vi "KioskDemoRight.vi"() -> ()   [LabVIEW 2023]
doc: "DESCRIPTION\nGeneral Application \n\nVERSION\nD1:00\nFirst Release To customer\nDD/MM/YYYY\n\nTemplate D2:01\nMade lighter and simpler\n14-04-2020"
uses:
  SubVIs/Controls/SetupModeState.ctl
  <vilib>/event_ctls.llb/eventsource.ctl
  SubVIs/Controls/DisplayQCommand.ctl
  SubVIs/Controls/QueueCommand.ctl
  SubVIs/Controls/DisplayMessage.ctl
  SubVIs/utilities/Error/ErrorCommand.ctl
  SubVIs/Controls/Transition.ctl
  <vilib>/Utility/miscctls.llb/LVBoundsTypeDef.ctl
  SubVIs/Buttons/ButtonCommands.ctl
  SubVIs/Buttons/MenuType.ctl
  <vilib>/Utility/miscctls.llb/LVPositionTypeDef.ctl
  SubVIs/Controls/Tab.ctl
  SubVIs/Controls/StateMessage.ctl
  SubVIs/Error/ErrorMessage.ctl
  SubVIs/utilities/Config/System Config Data Manager Parameter.ctl
  SubVIs/utilities/Config/ConfigCommand.ctl
panel:
  out "Selector ref out":refnum<vi>
  in  "Tab Control 2":enum32{"Page 3"}(tab)
  out "BGND ref out":refnum<vi>
  in  "exit":bool
  out "Application Directory":path
  in  "ButtonsMenu":enum32{"Page 1"}(tab)
  out "SubmenuVisible":bool
  out "State":T1=enum."Initialising"
  out "UI Output":string
  out "Menu Output":string
  in  "Stop":bool
  in  "Source":T2 items=["LabVIEW UI"=0, "ActiveX"=1, "User Event"=25]
  in  "Start":bool
  out "ErrorHandlingLoop":i32
  out "StateMachineLoop":i32
  out "UILoop":i32
  out "EventLoop":i32
  in  "Main Screen Tabs":enum32{"Main Screen"}(tab)
  out "Tab Control":T3(tab)
  in  "Error Loop":enum16{"Event Loop", "UI Q Loop", "State Loop"}(ring)
  in  "Generate Error":bool
  out "EngMode?":bool
  in  "Enter Password":string
  out "ConfigdB path":path
  in  "Home Button":bool
  in  "ErrorLog":bool
  in  "Clear Alarm":bool
  in  "ErrorLog":i32(listbox)
  out "Error":string
  out "ErrorIndicator":bool
  in  "ViewError":bool
  out "Version":string
  out "Time":string
  out "Status":string
  # "GenAppMain"
  # "Move to right and change sub menu"
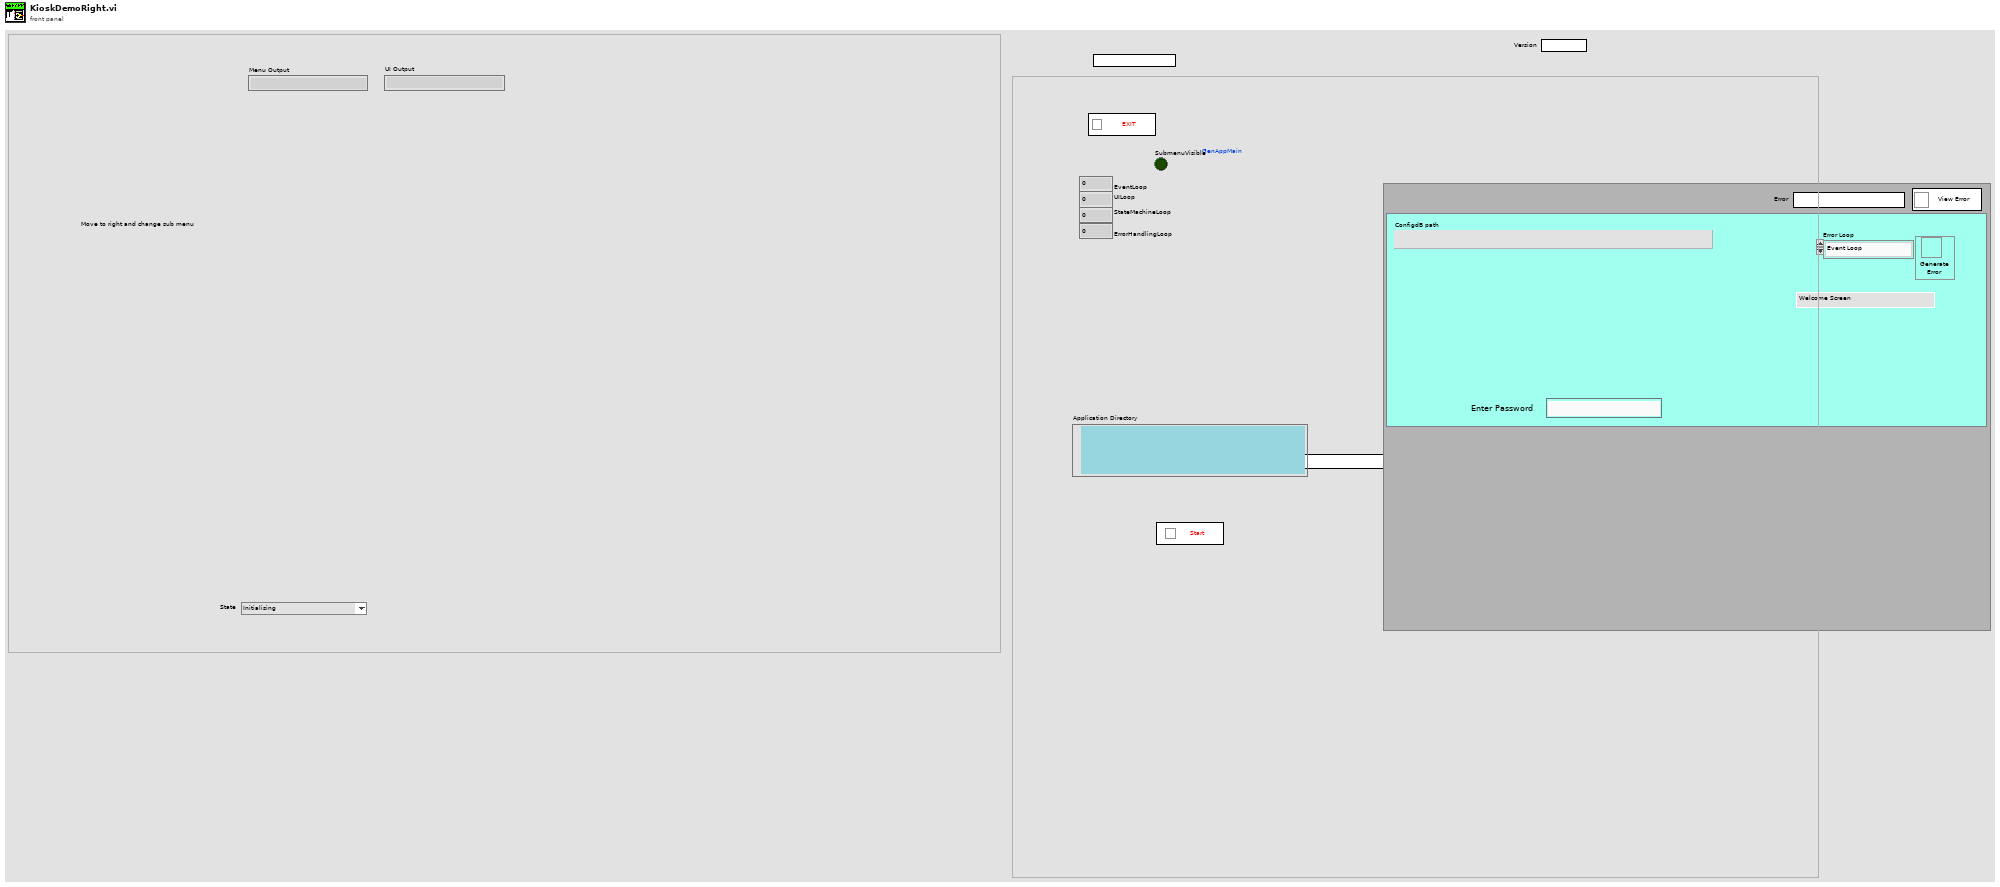
[diagram p1: front panel]
types:
  T1 = typedef "SetupModeState.ctl" = enum16{"No State - Error", "Initialising", "Idling", "Running", "Sorting Menu", "Resetting Menu", "Sorting Submenu", "Loading UI", "Erroring", "Exiting"}
  T2 = typedef "eventsource.ctl" = u32
  T3 = enum32{"Welcome Screen", "Eng Set Up", "Oppo Run Screen", "Eng Run Screen", "Test Report Screen", "Error"}
  T4 = typedef "DisplayQCommand.ctl" = enum16{"No Command - Error", "Initialise", "Get Q Reference", "Add Item to Bottom", "Add Item to Top", "Flush Q", "Dequeue", "Peek Next Element", "Close"}
  T5 = typedef "QueueCommand.ctl" = enum16{"No Command - Error", "Initialise", "Add to Bottom", "Add To Top", "Get Ref", "Close"}
  T6 = typedef "LVBoundsTypeDef.ctl" = cluster{"Width":u32, "Height":u32}
  T7 = typedef "ErrorCommand.ctl" = enum16{"No Command - Error", "Set to Dev Mode", "Set To Released Mode", "Set Error", "Log Error", "Throw Error", "Log & Throw Error", "Set Error Timed"}
  T8 = enum32{"invalid app kind", "Development System", "Run Time System", "Student Edition", "Embedded LabVIEW", "Evaluation", "Custom"}
  T9 = typedef "LVPositionTypeDef.ctl" = cluster{"Left":i32, "Top":i32}
  T10 = typedef "StateMessage.ctl" = cluster{"Transition":T11, "variant":variant}
  T11 = typedef "Transition.ctl" = enum16{"No Transition - Error", "Initialise", "Login", "Authenticate", "Log on Fail", "Login Success", "Logout", "Generate Error", "Start", "Stop", "Menu Button Pressed", "UI Button Pressed", "Exit"}
  T12 = typedef "DisplayMessage.ctl" = enum16{"No Message - Ignore", "Display Message", "Set Tab", "Set Status", "Add Error Message", "Clear Error History", "Generate Error", "Set Idling Display", "Set Running Display", "Set Subpanel Output", "Stop"}
  T13 = typedef "ErrorMessage.ctl" = enum16{"No Message - Ignore", "Display Message", "Stop"}
  T14 = typedef "ConfigCommand.ctl" = enum16{"No Command - Error", "Initialise Config SQLite", "Save Config", "Get Key", "Set Key", "Update Key", "Get Latest Config Data", "Get Config Data for Version", "Get Default Config Data"}
  T15 = typedef "System Config Data Manager Parameter.ctl" = enum16{"Eng Password", "DSN Connection", "User Password", "RunStatus", "InitialDataPath", "helpFilePath", "ErrorFilepath", "DatalogPath", "Hello"}
  T16 = typedef "Tab.ctl" = enum32{"Welcome Screen", "Eng Set Up", "Oppo Run Screen", "Eng Run Screen", "Test Report Screen", "Error"}
  T17 = typedef "lveventtype.ctl" = enum32{"Null", "Timeout", "Annotation Menu Selection", "Annotation Menu Selection?", "App Instance Close", "App Instance Close?", "Autoscale Range Change", "Bookmark Info Change", "Cell Edit", "Cell Edit?", "Cursor Grab", "Cursor Grab?", "Cursor Menu Selection", "Cursor Menu Selection?", "Cursor Move", "Cursor Release", "Data Change", "Direction Change", "Display State Change", "Drag Ended", "Drag Enter", "Drag Leave", "Drag Over", "Drag Source Update", "Drag Starting", "Drag Starting?", "Drop", "Exec State Change", "Key Down", "Key Down?", "Key Repeat", "Key Repeat?", "Key Up", "Listbox Double Click", "Menu Activation?", "Menu Selection (App)", "Menu Selection? (App)", "Menu Selection (User)", "Mouse Down", "Mouse Down?", "Mouse Enter", "Mouse Leave", "Mouse Move", "Mouse Up", "Mouse Wheel", "NI Security User Change (App)", "Pane Size", "Panel Close", "Panel Close?", "Panel Resize", "Plot Attribute Change", "Scale Range Change", "Shortcut Menu Activation?", "Shortcut Menu Selection (App)", "Shortcut Menu Selection? (App)", "Shortcut Menu Selection (User)", "Tree Double Click", "Tree Drag", "Tree Drag?", "Tree Drop", "Tree Drop?", "Tree Item Close", "Tree Item Close?", "Tree Item Open", "Tree Item Open?", "User Event", "Value Change"}
  T18 = typedef "MenuType.ctl" = enum16{"Main", "Simulation", "ME", "SF", "User Utilities", "Dev Tools"}
  T19 = typedef "ButtonCommands.ctl" = enum16{"No Command - Error", "Load Buttons", "Remove Buttons", "Get User Event"}
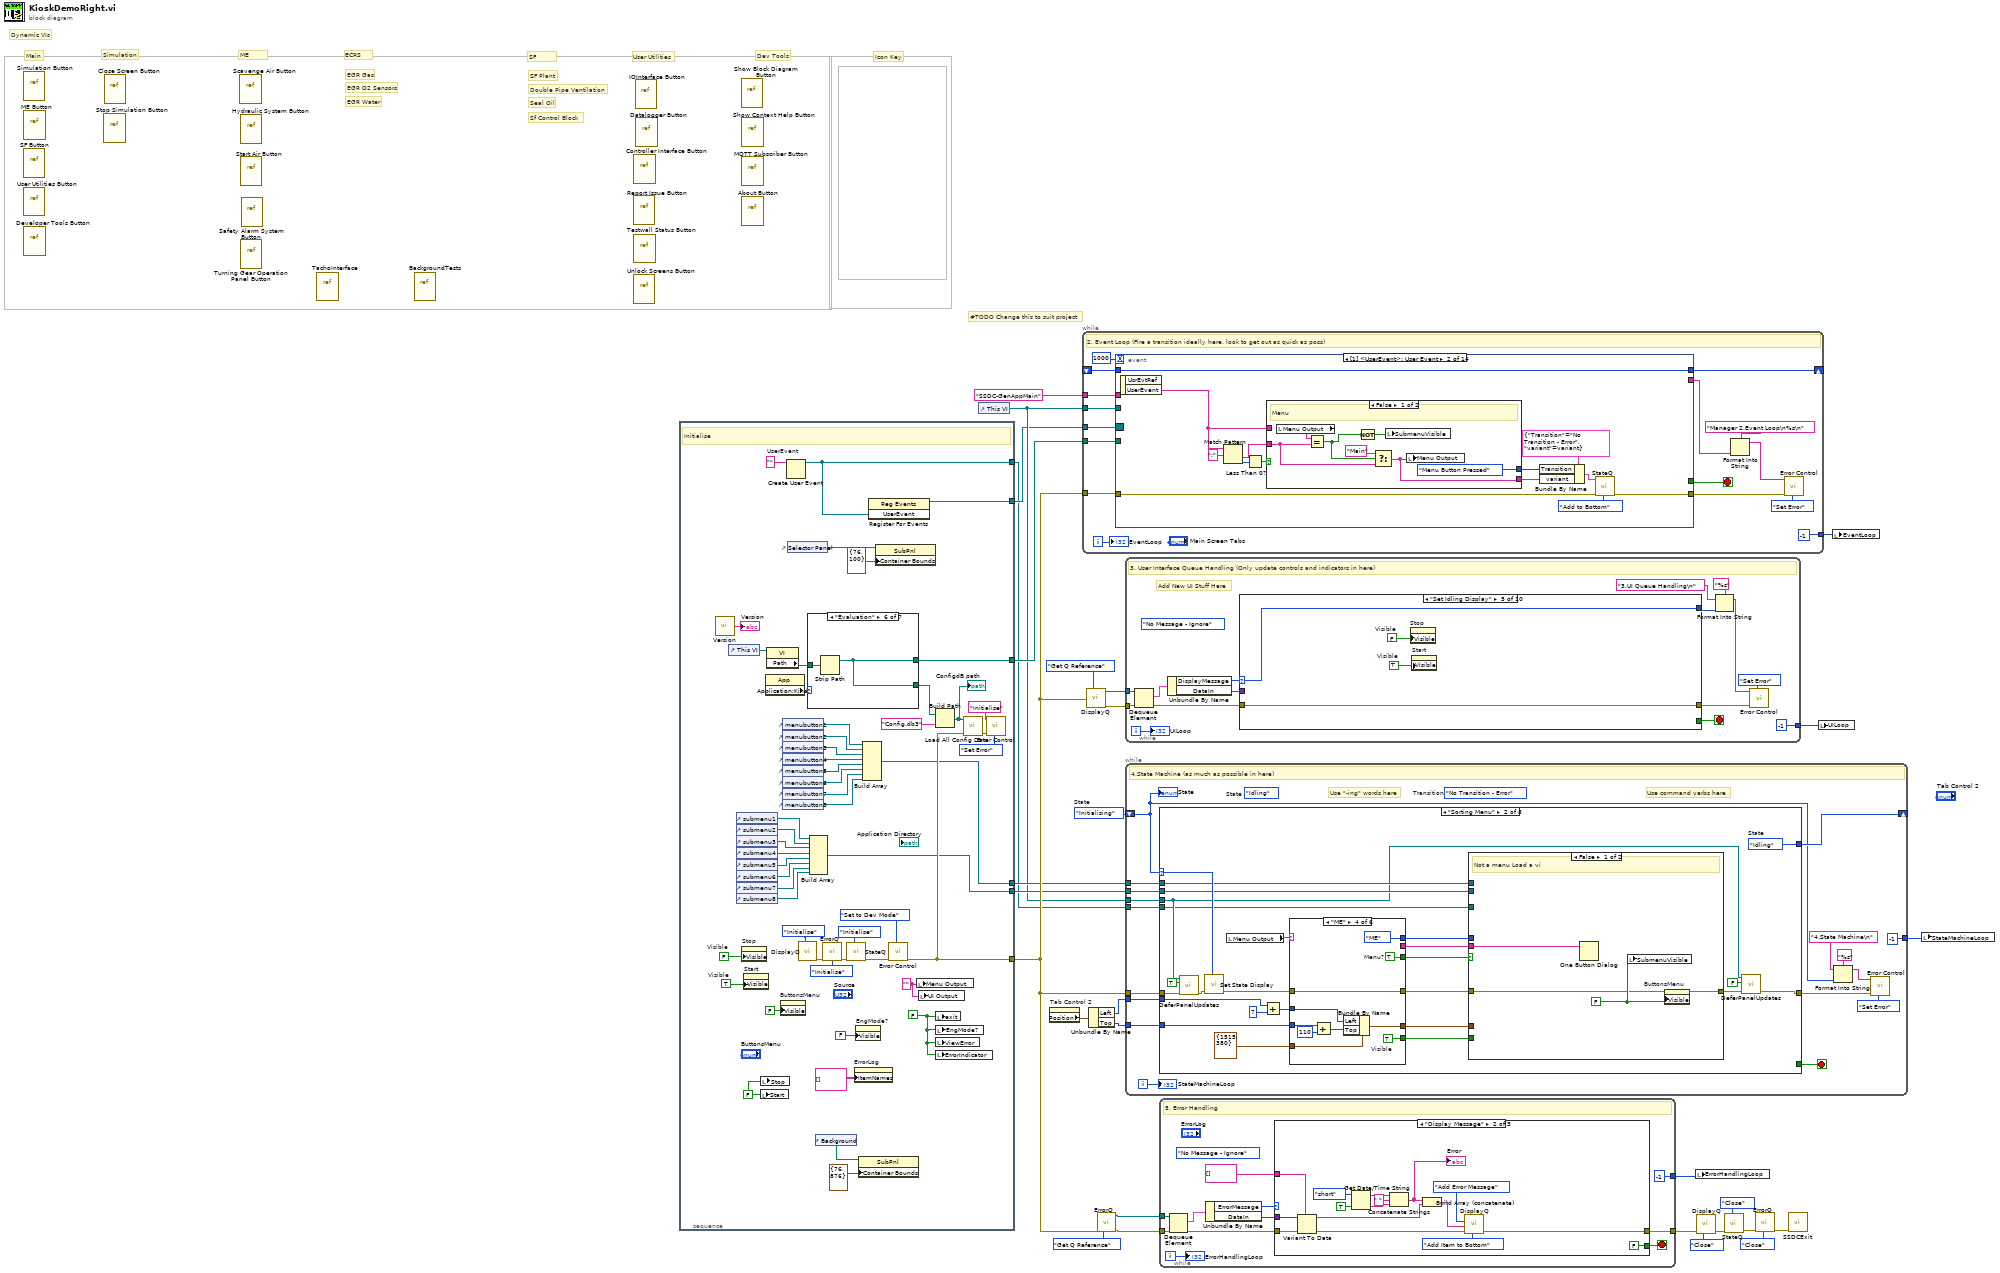
[diagram p0: block diagram]
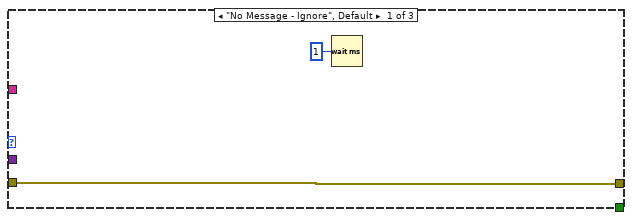
[diagram p2: hidden frame]
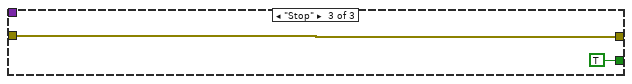
[diagram p3: hidden frame]
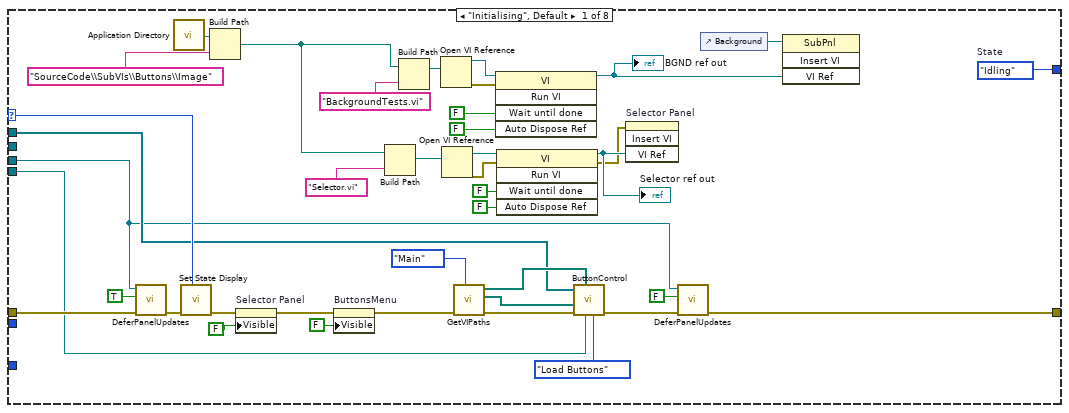
[diagram p4: hidden frame]
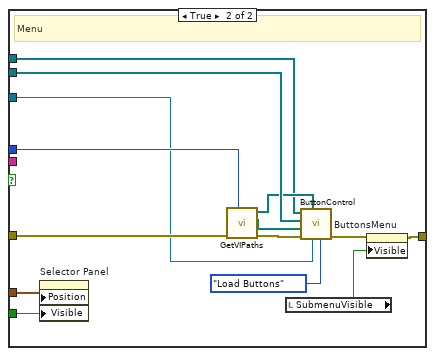
[diagram p5: hidden frame]
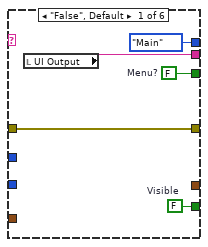
[diagram p6: hidden frame]
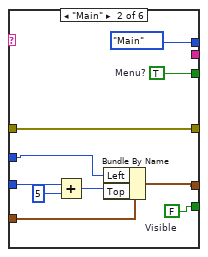
[diagram p7: hidden frame]
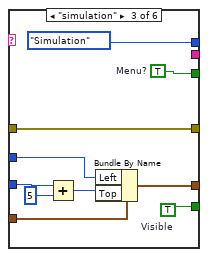
[diagram p8: hidden frame]
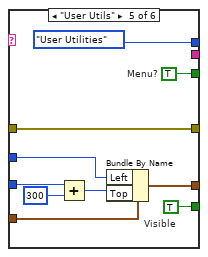
[diagram p9: hidden frame]
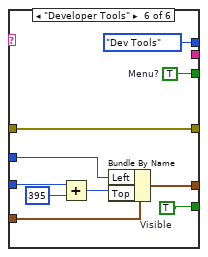
[diagram p10: hidden frame]
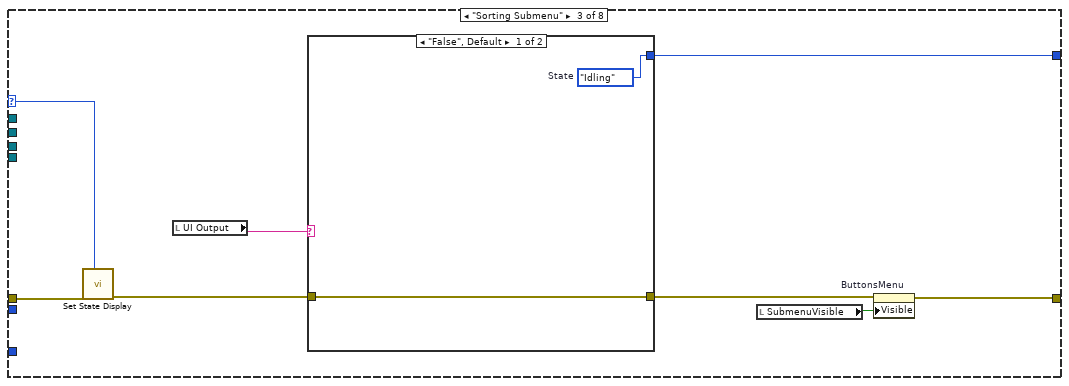
[diagram p11: hidden frame]
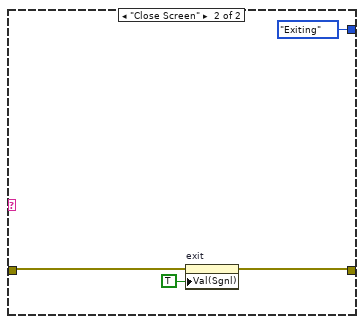
[diagram p12: hidden frame]
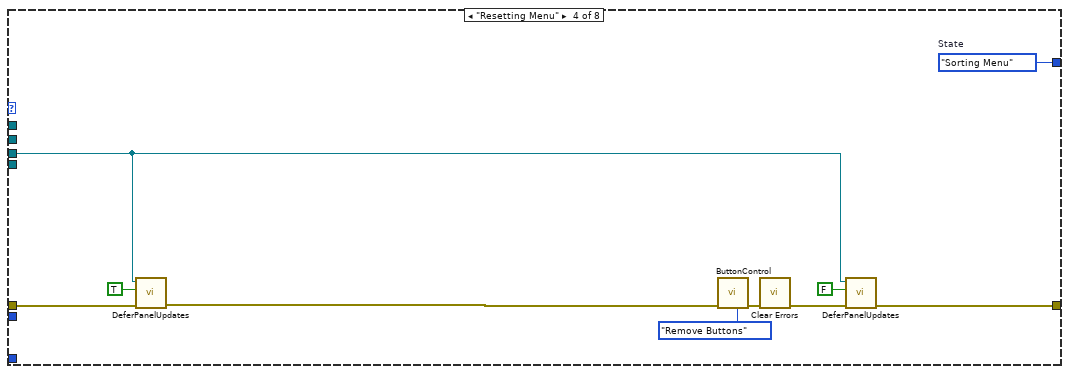
[diagram p13: hidden frame]
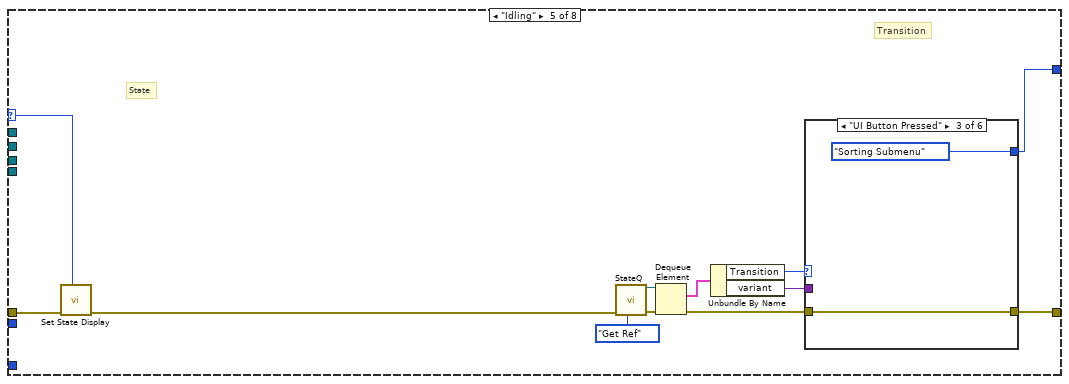
[diagram p14: hidden frame]
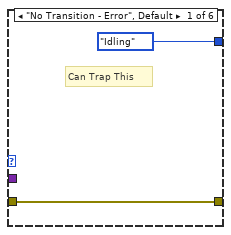
[diagram p15: hidden frame]
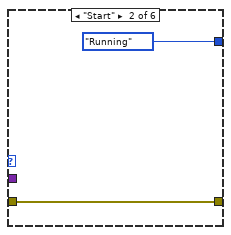
[diagram p16: hidden frame]
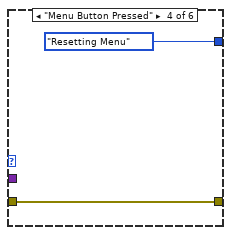
[diagram p17: hidden frame]
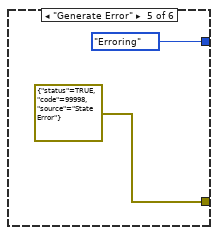
[diagram p18: hidden frame]
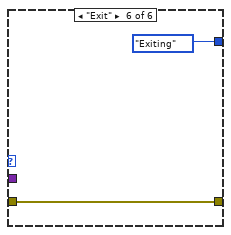
[diagram p19: hidden frame]
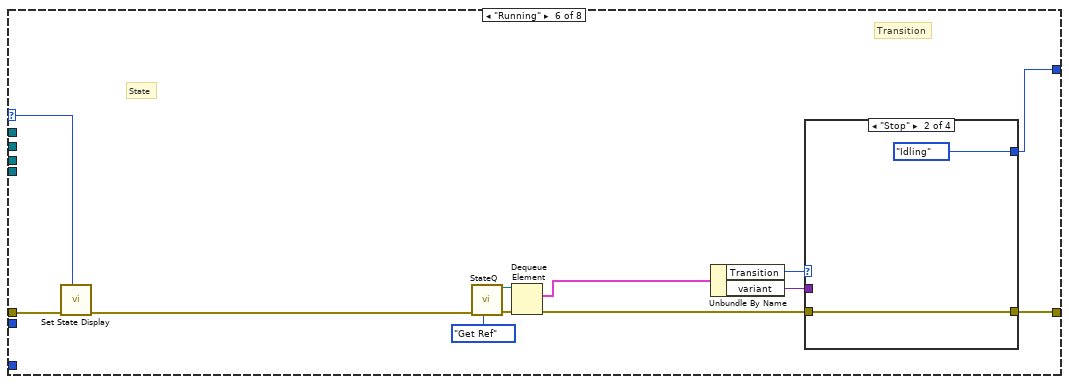
[diagram p20: hidden frame]
diagram:
  w29 = SetupModeState."Initialising"  # State
  # "Sf Control Block"
  # "Seal Oil"
  # "Double Pipe Ventilation"
  # "SF Plant"
  # "SF"
  # "EGR Water"
  # "EGR O2 Sensors"
  # "EGR Gas"
  # "ECRS"
  # "Dev Tools"
  # "User Utilities"
  # "Main"
  # "Simulation"
  # "ME"
  # "Dynamic VIs"
  # "#TODO Change this to suit project"
  # "Icon Key"
  n1 = vi-ref "Simulation Button.vi"() -> ()  [unwired: 1 out]
  n2 = vi-ref "SF Button.vi"() -> ()  [unwired: 1 out]
  n3 = vi-ref "User Utilities Button.vi"() -> ()  [unwired: 1 out]
  n4 = vi-ref "ME Button.vi"() -> ()  [unwired: 1 out]
  n5 = vi-ref "Developer Tools Button.vi"() -> ()  [unwired: 1 out]
  n6 = vi-ref "Stop Simulation Button.vi"() -> ()  [unwired: 1 out]
  n7 = vi-ref "Close Screen Button.vi"() -> ()  [unwired: 1 out]
  n8 = vi-ref "Scavenge Air Button.vi"() -> ()  [unwired: 1 out]
  n9 = vi-ref "Hydraulic System Button.vi"() -> ()  [unwired: 1 out]
  n10 = vi-ref "Start Air Button.vi"() -> ()  [unwired: 1 out]
  n11 = vi-ref "Turning Gear Operation Panel Button.vi"() -> ()  [unwired: 1 out]
  n12 = vi-ref "Safety Alarm System Button.vi"() -> ()  [unwired: 1 out]
  n13 = vi-ref "TachoInterface.vi"() -> ()  [unwired: 1 out]
  n14 = vi-ref "BackgroundTests.vi"() -> ()  [unwired: 1 out]
  n15 = vi-ref "Report Issue Button.vi"() -> ()  [unwired: 1 out]
  n16 = vi-ref "Unlock Screens Button.vi"() -> ()  [unwired: 1 out]
  n17 = vi-ref "Controller Interface Button.vi"() -> ()  [unwired: 1 out]
  n18 = vi-ref "Testwall Status Button.vi"() -> ()  [unwired: 1 out]
  n19 = vi-ref "IOInterface Button.vi"() -> ()  [unwired: 1 out]
  n20 = vi-ref "Datalogger Button.vi"() -> ()  [unwired: 1 out]
  n21 = stacked-sequence "1. Initialisation" {
    tunnel: [w60] -> w16
    tunnel: [w65] -> w24
    tunnel: [w49] -> w8
    tunnel: [w41] -> w7
    tunnel: [w35] -> w1
    tunnel: [w34] -> w5
    frame #0 {
      w36 = ""  # UserEvent
      w39 = "" ("Menu Output")
      w58 = FALSE  # Visible
      w57 = TRUE  # Visible
      w63 = FALSE ("Stopped")
      w59 = FALSE ("Start")
      # "Initialise"
      n22 = call "Version.vi"() -> ("Version"=→"Version":string)  [unwired: 5 in]
      n23 = control-ref of="This VI"() -> (w76:refnum<vi>)
      n24 = control-ref of="submenu1"() -> (w48:refnum<vi>)
      n25 = control-ref of="submenu2"() -> (w47:refnum<vi>)
      n26 = control-ref of="submenu3"() -> (w46:refnum<vi>)
      n27 = control-ref of="submenu4"() -> (w45:refnum<vi>)
      n28 = control-ref of="submenu5"() -> (w44:refnum<vi>)
      n29 = control-ref of="submenu6"() -> (w43:refnum<vi>)
      n30 = control-ref of="submenu7"() -> (w42:refnum<vi>)
      n31 = control-ref of="submenu8"() -> (w38:refnum<vi>)
      n32 = property on="Stop" class="Bool (strict)"("Visible"=w58) -> ()  [unwired: 2 in, 2 out]
      n33 = property on="Start" class="Bool (strict)"("Visible"=w57) -> ()  [unwired: 2 in, 2 out]
      n34 = local write "Start"(w59) -> ()
      n35 = local write "Stop"(w59) -> ()
      n36 = property class="App"() -> ("Application:Kind"=w75:T8)  [unwired: 2 in, 2 out]
      n37 = property class="VI"(reference=w76) -> ("Path"=w77:path)  [unwired: 1 in, 2 out]
      n38 = property on="ButtonsMenu" class="TabCtl (strict)"("Visible"=FALSE) -> ()  [unwired: 2 in, 2 out]
      n39 = control-ref of="menubutton1"() -> (w51:refnum<vi>)
      n40 = control-ref of="menubutton2"() -> (w50:refnum<vi>)
      n41 = control-ref of="menubutton3"() -> (w56:refnum<vi>)
      n42 = control-ref of="menubutton4"() -> (w55:refnum<vi>)
      n43 = control-ref of="menubutton5"() -> (w54:refnum<vi>)
      n44 = control-ref of="menubutton6"() -> (w53:refnum<vi>)
      n45 = control-ref of="menubutton7"() -> (w52:refnum<vi>)
      n46 = control-ref of="menubutton8"() -> (w40:refnum<vi>)
      n47 = Create User Event(user event datatype=w36) -> (user event=w35:refnum<user-event>)  [unwired: 1 in, 1 out]
      n48 = control-ref of="Selector Panel"() -> (w31:refnum<vi>)
      n49 = call "DisplayQ.vi"("command"=DisplayQCommand."Initialise") -> ("error out"=w70:errorcluster)  [unwired: 4 in, 3 out]
      n50 = case shown="\"Evaluation\"" w75 {
        tunnel: w77 -> [w82 w84 w88 w91 w93 w95 w97]
        tunnel: [w82 w83 w87 w90 w92 w94 w96] -> w66
        tunnel: [w82 w83 w85 w90 w92 w94 w96] -> w65
        frame "invalid app kind", Default {
        }
        frame "Development System" {
          n51 = Strip Path(path=w84) -> (stripped path=w83:path)  [unwired: 1 out]
        }
        frame "Run Time System" {
          n52 = Strip Path(path=w88) -> (stripped path=w89:path)  [unwired: 1 out]
          n53 = Strip Path(path=w89) -> (stripped path=w85:path)  [unwired: 1 out]
          n54 = Build Path(base path=w85, name or relative path="data") -> (appended path=w87:path)
        }
        frame "Student Edition" {
          n55 = Strip Path(path=w91) -> (stripped path=w90:path)  [unwired: 1 out]
        }
        frame "Embedded LabVIEW" {
          n56 = Strip Path(path=w93) -> (stripped path=w92:path)  [unwired: 1 out]
        }
        frame "Evaluation" {
          n57 = Strip Path(path=w95) -> (stripped path=w94:path)  [unwired: 1 out]
        }
        frame "Custom" {
          n58 = Strip Path(path=w97) -> (stripped path=w96:path)  [unwired: 1 out]
        }
      }
      n59 = Build Array(w48, w47, w46, w45, w44, w43, w42, w38) -> (w41:refnum<vi>[])
      n60 = control-ref of="Background"() -> (w33:refnum<vi>)
      n61 = call "ErrorQ.vi"("command"=DisplayQCommand."Initialise", "error in (no error)"=w70) -> ("error out"=w71:errorcluster)  [unwired: 3 in, 3 out]
      n62 = call "StateQ.vi"("QueueCommand"=QueueCommand."Initialise", "error in (no error)"=w71) -> ("error out"=w61:errorcluster)  [unwired: 5 in, 1 out]
      n63 = property on="ErrorLog" class="MCListbox (strict)"("ItemNames"=string[][] [] ("Item Names")) -> ()  [unwired: 2 in, 2 out]
      n64 = property on="EngMode?" class="Bool (strict)"("Visible"=FALSE) -> ()  [unwired: 2 in, 2 out]
      n65 = property class="SubPnl"(reference=w33, "Container Bounds"=T6 {"Width"=76, "Height"=876}) -> ()  [unwired: 1 in, 2 out]
      n66 = Build Array(w51, w50, w56, w55, w54, w53, w52, w40) -> (w49:refnum<vi>[])
      n67 = register-events(w35) -> (reference out=w34:refnum<event-registration>)  [unwired: 2 in, 1 out]
      n68 = property class="SubPnl"(reference=w31, "Container Bounds"=T6 {"Width"=76, "Height"=100}) -> ()  [unwired: 1 in, 2 out]
      n69 = call "Error Control.vi"("Command"=ErrorCommand."Set to Dev Mode", "error in (no error)"=w61) -> ("error out"=w60:errorcluster)  [unwired: 6 in]
      n70 = local write "Menu Output"(w39) -> ()
      n71 = local write "UI Output"(w39) -> ()
      n72 = local write "exit"(w63) -> ()
      n73 = local write "ViewError"(w63) -> ()
      n74 = local write "ErrorIndicator"(w63) -> ()
      n75 = Build Path(base path=w66, name or relative path="Config.db3") -> (appended path=w78:path)
      "ConfigdB path" <- w78
      n76 = local write "EngMode?"(w63) -> ()
      n77 = call "Load All Config Data.vi"("error in (no error)"=w60, "path"=w78) -> ("error out"=w68:errorcluster)  [unwired: 5 in]
      n78 = call "Error Control.vi"("Command"=ErrorCommand."Set Error", "error in (no error)"=w68, "Source"="Initialise") -> ()  [unwired: 5 in, 1 out]
    }
  }
  n79 = vi-ref "Show Block Diagram Button.vi"() -> ()  [unwired: 1 out]
  n80 = vi-ref "Show Context Help Button.vi"() -> ()  [unwired: 1 out]
  n81 = vi-ref "MQTT Subscriber Button.vi"() -> ()  [unwired: 1 out]
  n82 = vi-ref "About Button.vi"() -> ()  [unwired: 1 out]
  n83 = control-ref of="This VI"() -> (w6:refnum<vi>)
  n84 = property on="Tab Control 2" class="TabCtl (strict)"() -> ("Position"=w4:T9)  [unwired: 2 in, 2 out]
  n85 = while "2. Event Loop" {
    tunnel: w16 -> [w110]
    shift-right: [w107] -> _
    shift-left: _ -> [w106]
    tunnel: w6 -> [w105]
    tunnel: [-1 ("ErrorHandlingLoop")] -> w25
    tunnel: w24 -> [w103]
    tunnel: "SSDC-GenAppMain" ("name or relative path") -> [w102]
    tunnel: w5 -> [w98]
    i -> [w113]
    stop <- w112 stop-if-true
    # "2. Event Loop (Fire a transition ideally here, look to get out as quick as poss)"
    n86 = event shown="[1] <UserEvent>: User Event" {
      selector: w98 -> [_ _ _ _ _ _ _ _ _ _ _ _ _ _]
      dyn-events: _ -> [_ _ _ _ _ _ _ _ _ _ _ _ _ _]
      timeout: 1000 -> [_ _ _ _ _ _ _ _ _ _ _ _ _ _]
      tunnel: [_ _ FALSE ("STOP?") _ TRUE ("STOP?") _ _ _ w219 _ _ _ _ _] -> w112
      tunnel: w110 -> [_ w122 w145 _ _ w177 w192 _ w216 w236 w254 w267 w290 _]
      tunnel: [_ w121 w145 _ _ w176 w191 _ w215 w235 w253 w266 w289 _] -> w108
      tunnel: ["Timeout" _ "Panel Close?" ("Event") w149 w156 w173 w187 w201 w210 w228 w247 w260 w283 w302] -> w99
      tunnel: [w116 w133 w144 w154 w159 w180 w194 w204 w218 w231 w252 w263 w291 w306] -> w107
      tunnel: w106 -> [w116 w133 w144 w154 w159 w180 w194 w204 w218 _ w252 w263 w291 w306]
      tunnel: w105 -> [_ _ _ _ _ _ _ _ w217 _ _ _ _ w305]
      tunnel: w103 -> [_ _ _ _ _ _ _ _ w214 _ _ _ _ _]
      tunnel: w102 -> [_ _ _ _ _ _ _ _ _ _ _ _ _ _]
      event Timeout {
        n87 = event-data() -> ()  [unwired: 1 in, 1 out]
        n88 = Get Date/Time String(want seconds? (F)=TRUE) -> (date string=w119:string, time string=w118:string)  [unwired: 2 in]
        n89 = Concatenate Strings(w119, " " ("string"), w118) -> (→"Time":string)
      }
      event User Event {
        n90 = event-data() -> ("UserEvent"=w123:string)  [unwired: 1 in, 1 out]
        n91 = Match Pattern(string=w123, regular expression=":") -> (after substring=w132:string, offset past match=w128:i32)  [unwired: 1 in, 2 out]
        n92 = Less Than 0?(x=w128) -> (x < 0?=w129:bool)
        n93 = case shown="False" w129 {
          tunnel: w132 -> [w137 _]
          tunnel: [Transition."Menu Button Pressed" ("Transition") Transition."UI Button Pressed" ("Transition")] -> w130
          tunnel: [w134 w141] -> w131
          tunnel: w123 -> [_ w141]
          frame False {
            # "Menu"
            n94 = local read "Menu Output"() -> (w139:string)
            n95 = Equal?(x=w139, y=w137) -> (x = y?=w136:bool)
            n96 = Not(x=w136) -> (.not. x?=w135:bool)
            n97 = Select(t="Main", s=w136, f=w137) -> (s? t:f=w134:string)
            n98 = local write "SubmenuVisible"(w135) -> ()
            n99 = local write "Menu Output"(w134) -> ()
          }
          frame True {
            # "UI"
            n100 = local write "UI Output"(w141) -> ()
          }
        }
        n101 = Bundle By Name(cluster=T10 {"Transition"=enum."No Transition - Error", "variant"=variant} ("output cluster"), "Transition"=w130, "variant"=w131) -> (w127:T10)
        n102 = call "StateQ.vi"("QueueCommand"=QueueCommand."Add to Bottom", "error in (no error)"=w122, "output cluster"=w127) -> ("error out"=w121:errorcluster)  [unwired: 4 in, 1 out]
      }
      event Panel Close? {
        n103 = event-data() -> ()  [unwired: 1 in, 1 out]
        n104 = property on="exit" class="Bool (strict)"("Val(Sgnl)"=TRUE ("Value (Signaling)")) -> ()  [unwired: 2 in, 2 out]
        n105 = event-data("Discard?"=TRUE) -> ()  [unwired: 1 in, 1 out]
      }
      event "ErrorLog": Value Change {
        n106 = event-data() -> ("CtlRef"=w151:refnum<vi>, "Type"=w150:T17)  [unwired: 1 in]
        n107 = call "CreateEventString.vi"("Type in"=w150, "Ctl Refnum"=w151) -> ("Event"=w149:string)  [unwired: 9 in]
        n108 = case shown="True" "ErrorLog" {
          tunnel: [_ FALSE] -> w152
          frame False {
          }
          frame True {
            n109 = call "ErrorLogDialog.vi"() -> ()  [unwired: 11 in, 1 out]
          }
        }
        n110 = local write "ErrorLog"(w152) -> ()
      }
      event "exit": Value Change {
        n111 = event-data() -> ("CtlRef"=w158:refnum<vi>, "Type"=w157:T17)  [unwired: 1 in]
        n112 = local write "Start"(FALSE ("Start")) -> ()
        n113 = call "CreateEventString.vi"("Type in"=w157, "Ctl Refnum"=w158) -> ("Event"=w156:string)  [unwired: 9 in]
        n114 = stacked-sequence {
          tunnel: [_ FALSE] -> w160
          frame #0 {
            n115 = call "StateQ.vi"("QueueCommand"=QueueCommand."Add To Top", "output cluster"=T10 {"Transition"=enum."Exit", "variant"=variant}) -> ("error out"=w167:errorcluster)  [unwired: 5 in, 1 out]
            n116 = call "ErrorQ.vi"("command"=DisplayQCommand."Add Item to Top", "error in (no error)"=w167, "ErrorMessage"=ErrorMessage."Stop") -> ("error out"=w164:errorcluster)  [unwired: 2 in, 3 out]
            n117 = call "DisplayQ.vi"("command"=DisplayQCommand."Add Item to Top", "error in (no error)"=w164, "DisplayMessage"=DisplayMessage."Stop") -> ()  [unwired: 2 in, 4 out]
          }
          frame #1 {
            n118 = Wait (ms)(milliseconds to wait=u32 500) -> ()  [unwired: 1 out]
          }
        }
        n119 = local write "exit"(w160) -> ()
      }
      event "Start": Value Change {
        n120 = event-data() -> ("CtlRef"=w175:refnum<vi>, "Type"=w174:T17)  [unwired: 1 in]
        n121 = call "CreateEventString.vi"("Type in"=w174, "Ctl Refnum"=w175) -> ("Event"=w173:string)  [unwired: 9 in]
        n122 = case shown="True" "Start" {
          tunnel: [_ FALSE ("Start")] -> w178
          tunnel: w177 -> [w181 w183]
          tunnel: [w181 w182] -> w176
          frame False {
          }
          frame True {
            n123 = call "StateQ.vi"("QueueCommand"=QueueCommand."Add To Top", "error in (no error)"=w183, "output cluster"=T10 {"Transition"=enum."Start", "variant"=variant}) -> ("error out"=w182:errorcluster)  [unwired: 4 in, 1 out]
          }
        }
        n124 = local write "Start"(w178) -> ()
      }
      event "Stop": Value Change {
        n125 = event-data() -> ("CtlRef"=w189:refnum<vi>, "Type"=w188:T17)  [unwired: 1 in]
        n126 = call "CreateEventString.vi"("Type in"=w188, "Ctl Refnum"=w189) -> ("Event"=w187:string)  [unwired: 9 in]
        n127 = case shown="True" "Stop" {
          tunnel: [_ FALSE ("Start")] -> w193
          tunnel: w192 -> [w195 w197]
          tunnel: [w195 w196] -> w191
          frame False {
          }
          frame True {
            n128 = call "StateQ.vi"("QueueCommand"=QueueCommand."Add To Top", "error in (no error)"=w197, "output cluster"=T10 {"Transition"=enum."Stop", "variant"=variant}) -> ("error out"=w196:errorcluster)  [unwired: 4 in, 1 out]
          }
        }
        n129 = local write "Stop"(w193) -> ()
      }
      event "Enter Password": Value Change {
        n130 = event-data() -> ("CtlRef"=w203:refnum<vi>, "Type"=w202:T17)  [unwired: 1 in]
        n131 = call "CreateEventString.vi"("Type in"=w202, "Ctl Refnum"=w203) -> ("Event"=w201:string)  [unwired: 9 in]
        n132 = call "SQLiteConfig.vi"("ConfigCommand"=ConfigCommand."Get Key", "Parameter"=System_Config_Data_Manager_Parameter."Eng Password") -> ("KeyData"=w205:string)  [unwired: 3 in, 3 out]
        n133 = Equal?(x=w205, y="Enter Password") -> (x = y?=w209:bool)
        "EngMode?" <- w209
        n134 = property on="EngMode?" class="Bool (strict)"("Visible"=w209) -> ()  [unwired: 2 in, 2 out]
      }
      event Menu Selection (User) {
        n135 = event-data() -> ("Type"=w212:T17, "ItemTag"=w211:string)  [unwired: 1 in]
        n136 = Format Into String(format string="\"Menu\":%s:%s", w212, w211) -> (resulting string=w210:string)  [unwired: 2 in, 1 out]
        n137 = case shown="\"About\"" w211 {
          tunnel: [_ FALSE _ _] -> w219
          tunnel: w217 -> [_ _ _ w227]
          tunnel: w216 -> [w220 w221 w224 w225]
          tunnel: [w220 w221 w224 w225] -> w215
          tunnel: w214 -> [_ _ _ _]
          frame "False", Default {
          }
          frame "Exit" {
            n138 = property on="exit" class="Bool (strict)"("Val(Sgnl)"=TRUE ("Value (Signaling)")) -> ()  [unwired: 2 in, 2 out]
          }
          frame "Configuration" {
            n139 = call "ConfigSQLiteSettingDialog.vi"() -> ()  [unwired: 1 in]
          }
          frame "About" {
            n140 = property class="VI"(reference=w227) -> ("Description"=w226:string)  [unwired: 1 in, 2 out]
            n141 = call "AboutScreen.vi"("Version Info. In"=w226) -> ()  [unwired: 11 in]
          }
        }
      }
      event "ViewError": Value Change {
        n142 = event-data() -> ("CtlRef"=w229:refnum<vi>, "Type"=w230:T17)  [unwired: 1 in]
        n143 = local read "Tab Control"() -> (w232:T3)
        n144 = call "CreateEventString.vi"("Type in"=w230, "Ctl Refnum"=w229) -> ("Event"=w228:string)  [unwired: 9 in]
        n145 = case shown="True" "ViewError" {
          tunnel: w236 -> [w239 w243]
          tunnel: [w239 w242] -> w235
          tunnel: [FALSE FALSE] -> w233
          tunnel: w232 -> [w237 w240]
          tunnel: [w237 w240] -> w231
          frame False {
          }
          frame True {
            n146 = call "DisplayQ.vi"("command"=DisplayQCommand."Add Item to Bottom", "error in (no error)"=w243, "DataIn"=Tab."Error" ("Tab Control"), "DisplayMessage"=DisplayMessage."Set Tab") -> ("error out"=w242:errorcluster)  [unwired: 1 in, 3 out]
          }
        }
        n147 = local write "ViewError"(w233) -> ()
      }
      event "Clear Alarm": Value Change {
        n148 = event-data() -> ("CtlRef"=w248:refnum<vi>, "Type"=w249:T17)  [unwired: 1 in]
        n149 = call "CreateEventString.vi"("Type in"=w249, "Ctl Refnum"=w248) -> ("Event"=w247:string)  [unwired: 9 in]
        n150 = case shown="True" "Clear Alarm" {
          tunnel: w254 -> [w256 w258]
          tunnel: [w256 w258] -> w253
          tunnel: [FALSE FALSE] -> w250
          frame False {
          }
          frame True {
            n151 = local write "ErrorIndicator"(FALSE ("ErrorIndicator")) -> ()
          }
        }
        n152 = local write "Clear Alarm"(w250) -> ()
      }
      event "Home Button": Value Change {
        n153 = event-data() -> ("CtlRef"=w262:refnum<vi>, "Type"=w261:T17)  [unwired: 1 in]
        n154 = call "CreateEventString.vi"("Type in"=w261, "Ctl Refnum"=w262) -> ("Event"=w260:string)  [unwired: 9 in]
        n155 = case shown="True" "Home Button" {
          tunnel: w267 -> [w269 w274]
          tunnel: [w269 w273] -> w266
          tunnel: [FALSE FALSE] -> w265
          tunnel: w263 -> [_ w271]
          frame False {
          }
          frame True {
            n156 = case shown="\"Error\"" w271 {
              tunnel: [Tab."Welcome Screen" ("Tab Control") Tab."Oppo Run Screen" ("Tab Control") Tab."Eng Run Screen" ("Tab Control") Tab."Test Report Screen" ("Tab Control") Tab."Error" ("Tab Control") Tab."Eng Run Screen" ("Tab Control")] -> w270
              frame "Welcome Screen" {
              }
              frame "Oppo Run Screen" {
              }
              frame "Eng Run Screen" {
              }
              frame "Test Report Screen" {
              }
              frame "Error" {
              }
              frame "Eng Set Up" {
              }
            }
            n157 = call "DisplayQ.vi"("command"=DisplayQCommand."Add Item to Bottom", "error in (no error)"=w274, "DataIn"=w270, "DisplayMessage"=DisplayMessage."Set Tab") -> ("error out"=w273:errorcluster)  [unwired: 1 in, 3 out]
          }
        }
        n158 = local write "Home Button"(w265) -> ()
      }
      event "Generate Error": Value Change {
        n159 = event-data() -> ("CtlRef"=w285:refnum<vi>, "Type"=w284:T17)  [unwired: 1 in]
        n160 = call "CreateEventString.vi"("Type in"=w284, "Ctl Refnum"=w285) -> ("Event"=w283:string)  [unwired: 9 in]
        n161 = case shown="\"UI Q Loop\"" "Error Loop" {
          tunnel: w290 -> [_ w294 w299]
          tunnel: [errorcluster {"status"=TRUE, "code"=99999, "source"="Random Event Error"} ("error out") w293 w300] -> w289
          tunnel: "Generate Error" -> [_ _ _]
          tunnel: [_ _ FALSE] -> w286
          frame "Event Loop", Default {
          }
          frame "UI Q Loop" {
            n162 = call "DisplayQ.vi"("command"=DisplayQCommand."Add Item to Bottom", "error in (no error)"=w294, "DisplayMessage"=DisplayMessage."Generate Error") -> ("error out"=w293:errorcluster)  [unwired: 2 in, 3 out]
          }
          frame "State Loop" {
            n163 = call "StateQ.vi"("QueueCommand"=QueueCommand."Add to Bottom", "error in (no error)"=w299, "output cluster"=T10 {"Transition"=enum."Generate Error", "variant"=variant}) -> ("error out"=w300:errorcluster)  [unwired: 4 in, 1 out]
          }
        }
        n164 = local write "Generate Error"(w286) -> ()
      }
      event "Version": Mouse Down {
        n165 = event-data() -> ("CtlRef"=w304:refnum<vi>, "Type"=w303:T17)  [unwired: 1 in]
        n166 = call "CreateEventString.vi"("Type in"=w303, "Ctl Refnum"=w304) -> ("Event"=w302:string)  [unwired: 9 in]
        n167 = property class="VI"(reference=w305) -> ("Description"=w307:string)  [unwired: 1 in, 2 out]
        n168 = call "VIDescription.vi"("VersionData In"=w307) -> ()  [unwired: 10 in, 1 out]
      }
    }
    n169 = Format Into String(format string="Manager 2.Event Loop\n%s\n", w99) -> (resulting string=w100:string)  [unwired: 2 in, 1 out]
    n170 = call "Error Control.vi"("Command"=ErrorCommand."Set Error", "error in (no error)"=w108, "Source"=w100) -> ()  [unwired: 5 in, 1 out]
    "EventLoop" <- w113
  }
  n171 = call "DisplayQ.vi"("command"=DisplayQCommand."Get Q Reference", "error in (no error)"=w16) -> ("error out"=w18:errorcluster, "queue out"=w19:refnum<queue>)  [unwired: 3 in, 2 out]
  n172 = Unbundle By Name(w4) -> ("Left"=w3:i32, "Top"=w2:i32)
  n173 = call "ErrorQ.vi"("command"=DisplayQCommand."Get Q Reference", "error in (no error)"=w16) -> ("error out"=w21:errorcluster, "queue out"=w22:refnum<queue>)  [unwired: 3 in, 2 out]
  n174 = while "3. User Interface Queue Handling" {
    tunnel: w18 -> [w322]
    tunnel: w19 -> [w321]
    tunnel: [-1 ("ErrorHandlingLoop")] -> w26
    i -> [w313]
    stop <- w314 stop-if-true
    (unwired) DisplayMessage."No Message - Ignore" ("DisplayMessage")
    # "Add New UI Stuff Here"
    # "3. User Interface Queue Handling (Only update controls and indicators in here)"
    n175 = Dequeue Element(queue=w321, error in (no error)=w322) -> (element=w320:cluster{"DisplayMessage":T12, "DataIn":variant}, error out=w317:errorcluster)  [unwired: 1 in, 2 out]
    n176 = Unbundle By Name(w320) -> ("DisplayMessage"=w318:T12, "DataIn"=w319:variant)
    n177 = case shown="\"Set Idling Display\"" w318 {
      selector: w318 -> [w323 w326 w329 w344 w351 w355 w359 w361 w363 w383]
      tunnel: w319 -> [_ _ w338 w347 _ _ _ _ w367 w369]
      tunnel: w317 -> [w324 w328 w331 w346 w350 w354 w358 _ w365 w370]
      tunnel: [w324 w328 w330 w345 w350 w354 w358 errorcluster {"status"=TRUE, "code"=99997, "source"="UI Error"} ("error out") w364 w368] -> w316
      tunnel: [_ TRUE ("STOP?") _ _ _ _ _ _ _ _] -> w314
      tunnel: [w323 w326 w329 w344 w351 w355 w359 w361 w363 w383] -> w312
      frame "No Message - Ignore", Default {
        n178 = Wait (ms)(milliseconds to wait=u32 1) -> ()  [unwired: 1 out]
      }
      frame "Stop" {
      }
      frame "Display Message" {
        n179 = Variant To Data(error in=w331, type="" ("data"), Variant=w338) -> (data=w334:string, error out=w330:errorcluster)
        n180 = local read "State"() -> (w336:T1)
        n181 = Format Into String(w336) -> (resulting string=w335:string)  [unwired: 3 in, 1 out]
        n182 = Concatenate Strings(w335, " - " ("string"), w334) -> (→"Status":string)
      }
      frame "Add Error Message" {
        n183 = property on="ErrorLog" class="MCListbox (strict)"() -> ("ItemNames"=w342:string[][])  [unwired: 2 in, 2 out]
        n184 = Variant To Data(error in=w346, type=string[] [], Variant=w347) -> (data=w341:string[], error out=w345:errorcluster)
        n185 = Build Array (concatenate)(w342, w341) -> (w339:string[][])
        n186 = property on="ErrorLog" class="MCListbox (strict)"("ItemNames"=w339) -> ()  [unwired: 2 in, 2 out]
        "ErrorIndicator" <- TRUE ("ErrorIndicator")
      }
      frame "Set Idling Display" {
        w348 = FALSE  # Visible
        w349 = TRUE  # Visible
        n187 = property on="Stop" class="Bool (strict)"("Visible"=w348) -> ()  [unwired: 2 in, 2 out]
        n188 = property on="Start" class="Bool (strict)"("Visible"=w349) -> ()  [unwired: 2 in, 2 out]
      }
      frame "Set Running Display" {
        w352 = TRUE  # Visible
        w353 = FALSE  # Visible
        n189 = property on="Stop" class="Bool (strict)"("Visible"=w352) -> ()  [unwired: 2 in, 2 out]
        n190 = property on="Start" class="Bool (strict)"("Visible"=w353) -> ()  [unwired: 2 in, 2 out]
      }
      frame "Clear Error History" {
        n191 = property on="ErrorLog" class="MCListbox (strict)"("ItemNames"=string[][] []) -> ()  [unwired: 2 in, 2 out]
        n192 = local write "ErrorIndicator"(FALSE ("ErrorIndicator")) -> ()
      }
      frame "Generate Error" {
      }
      frame "Set Tab" {
        n193 = Variant To Data(error in=w365, type=Tab."Eng Run Screen" ("Tab Control"), Variant=w367) -> (data=→"Tab Control":T16, error out=w364:errorcluster)
      }
      frame "Set Subpanel Output" {
        n194 = Variant To Data(error in=w370, type="", Variant=w369) -> (data=w382:string, error out=w375:errorcluster)
        n195 = Match Pattern(string=w382, regular expression=":") -> (after substring=w381:string, offset past match=w377:i32)  [unwired: 1 in, 2 out]
        n196 = Less Than 0?(x=w377) -> (x < 0?=w378:bool)
        n197 = case shown="False" w378 {
          tunnel: w381 -> [w387 _]
          tunnel: [Transition."Menu Button Pressed" ("Transition") Transition."UI Button Pressed" ("Transition")] -> w379
          tunnel: [w386 w391] -> w380
          tunnel: w382 -> [_ w391]
          frame False {
            # "Menu"
            n198 = local read "Menu Output"() -> (w389:string)
            n199 = Equal?(x=w389, y=w387) -> (x = y?=w385:bool)
            n200 = Not(x=w385) -> (.not. x?=→"SubmenuVisible":bool)
            n201 = Select(t="Main", s=w385, f=w387) -> (s? t:f=w386:string)
            "Menu Output" <- w386
          }
          frame True {
            # "UI"
            "UI Output" <- w391
          }
        }
        n202 = Bundle By Name(cluster=T10 {"Transition"=enum."No Transition - Error", "variant"=variant} ("output cluster"), "Transition"=w379, "variant"=w380) -> (w376:T10)
        n203 = call "StateQ.vi"("QueueCommand"=QueueCommand."Add to Bottom", "error in (no error)"=w375, "output cluster"=w376) -> ("error out"=w368:errorcluster)  [unwired: 4 in, 1 out]
      }
    }
    n204 = Format Into String(format string="%s", initial string="3.UI Queue Handling\n", w312) -> (resulting string=w311:string)  [unwired: 1 in, 1 out]
    n205 = call "Error Control.vi"("Command"=ErrorCommand."Set Error", "error in (no error)"=w316, "Source"=w311) -> ()  [unwired: 5 in, 1 out]
    "UILoop" <- w313
  }
  n206 = while {
    shift-right: [w407] -> _
    shift-left: w29 -> [w403]
    tunnel: w16 -> [w408]
    tunnel: [-1 ("ErrorHandlingLoop")] -> w27
    tunnel: w8 -> [w398]
    tunnel: w7 -> [w397]
    tunnel: w6 -> [w396]
    tunnel: w3 -> [w395]
    tunnel: w2 -> [w394]
    tunnel: w1 -> [w393]
    i -> [w406]
    stop <- w409 stop-if-true
    (unwired) SetupModeState."Idling"  # State
    (unwired) Transition."No Transition - Error"  # Transition
    # "Use command verbs here"
    # "Use \"-ing\" words here"
    # "4.State Machine (as much as possible in here)"
    n207 = case shown="\"Sorting Menu\"" w403 {
      selector: w403 -> [w440 w473 w555 _ w582 w606 w616 w640]
      tunnel: [_ _ _ _ _ _ _ TRUE] -> w409
      tunnel: w408 -> [w439 w465 w554 w566 w583 w607 w620 w638]
      tunnel: [w449 w474 w548 w571 w573 w597 w619 SetupModeState."No State - Error" ("State 2")] -> w407
      tunnel: [w438 w460 w553 w565 w574 w598 w618 w637] -> w404
      tunnel: w398 -> [w437 w468 _ _ _ _ _ _]
      tunnel: w397 -> [_ w467 _ _ _ _ _ _]
      tunnel: w396 -> [w436 w459 _ w564 _ _ _ w639]
      tunnel: w395 -> [_ w452 _ _ _ _ _ _]
      tunnel: w394 -> [_ w451 _ _ _ _ _ _]
      tunnel: w393 -> [w410 w450 _ _ _ _ _ _]
      frame "Initialising", Default {
        w449 = SetupModeState."Idling"  # State
        n208 = call "DeferPanelUpdates.vi"("error in (no error)"=w439, "Defer Panel Updates"=TRUE, "VI in"=w436) -> ("error out"=w443:errorcluster)  [unwired: 8 in]
        n209 = call <vilib>:"Application Directory.vi"() -> ("Application Directory"=w425:path)
        n210 = call "Set State Display.vi"("State"=w440, "error in (no error)"=w443) -> ("error out"=w413:errorcluster)  [unwired: 6 in]
        n211 = Build Path(base path=w425, name or relative path="SourceCode\\SubVIs\\Buttons\\Image") -> (appended path=w418:path)
        n212 = property on="Selector Panel" class="SubPnl"(error in=w413, "Visible"=FALSE) -> (error out=w412:errorcluster)  [unwired: 1 in, 1 out]
        n213 = property on="ButtonsMenu" class="TabCtl (strict)"(error in=w412, "Visible"=FALSE) -> (error out=w433:errorcluster)  [unwired: 1 in, 1 out]
        n214 = Build Path(base path=w418, name or relative path="Selector.vi") -> (appended path=w419:path)
        n215 = Build Path(base path=w418, name or relative path="BackgroundTests.vi") -> (appended path=w426:path)
        n216 = Open VI Reference(vi path=w426) -> (vi reference=w429:refnum<vi>, error out=w430:errorcluster)  [unwired: 5 in]
        n217 = Open VI Reference(vi path=w419) -> (vi reference=w422:refnum<vi>, error out=w421:errorcluster)  [unwired: 5 in]
        n218 = call "GetVIPaths.vi"("MenuType"=MenuType."Main", "error in (no error)"=w433) -> ("error out"=w448:errorcluster, "SubMenu VIs"=w446:path[], "Menu VIs"=w445:path[])  [unwired: 4 in]
        n219 = invoke class="VI" method="Run VI"(reference=w429, error in=w430, "Wait until done"=FALSE ("Wait Until Done"), "Auto Dispose Ref"=FALSE ("Auto Dispose Reference")) -> (reference out=w428:refnum<vi>)  [unwired: 1 in, 4 out]
        "BGND ref out" <- w428
        n220 = invoke class="VI" method="Run VI"(reference=w422, error in=w421, "Wait until done"=FALSE ("Wait Until Done"), "Auto Dispose Ref"=FALSE ("Auto Dispose Reference")) -> (reference out=w417:refnum<vi>, error out=w414:errorcluster)  [unwired: 1 in, 3 out]
        "Selector ref out" <- w417
        n221 = call "ButtonControl.vi"("SubPanel Command"=ButtonCommands."Load Buttons", "user event in"=w410, "MenuButtons"=w445, "error in (no error)"=w448, "SubMenuButtons"=w446, "MenuButtonPanels"=w437) -> ("error out"=w441:errorcluster)  [unwired: 3 in, 1 out]
        n222 = invoke on="Selector Panel" class="SubPnl" method="Insert VI"(error in=w414, "VI Ref"=w417) -> ()  [unwired: 2 in, 4 out]
        n223 = call "DeferPanelUpdates.vi"("error in (no error)"=w441, "Defer Panel Updates"=FALSE, "VI in"=w436) -> ("error out"=w438:errorcluster)  [unwired: 8 in]
        n224 = control-ref of="Background"() -> (w423:refnum<vi>)
        n225 = invoke on="Invoke Node" class="SubPnl" method="Insert VI"(reference=w423, "VI Ref"=w428) -> ()  [unwired: 2 in, 4 out]
      }
      frame "Sorting Menu" {
        w474 = SetupModeState."Idling"  # State
        n226 = call "DeferPanelUpdates.vi"("error in (no error)"=w465, "Defer Panel Updates"=TRUE, "VI in"=w459) -> ("error out"=w464:errorcluster)  [unwired: 8 in]
        n227 = call "Set State Display.vi"("State"=w473, "error in (no error)"=w464) -> ("error out"=w463:errorcluster)  [unwired: 6 in]
        n228 = local read "Menu Output"() -> (w472:string)
        n229 = Add(x=w452, y=7) -> (x+y=w455:i32)
        n230 = case shown="\"ME\"" w472 {
          tunnel: w463 -> [w497 w507 w517 w527 w537 w547]
          tunnel: [w497 w507 w517 w527 w537 w547] -> w458
          tunnel: [MenuType."Main" ("MenuType") MenuType."Main" ("MenuType") MenuType."Simulation" ("MenuType") MenuType."ME" ("MenuType") MenuType."User Utilities" ("MenuType") MenuType."Dev Tools" ("MenuType")] -> w471
          tunnel: [w496 w506 w516 w526 w536 w546] -> w470
          tunnel: [w494 _ _ _ _ _] -> w469
          tunnel: w451 -> [_ w501 w510 w519 w529 w539]
          tunnel: T9 {"Left"=1515, "Top"=380} ("Position") -> [_ w500 w514 w521 w531 w541]
          tunnel: w455 -> [_ w502 w513 w522 w532 w542]
          tunnel: [_ w499 w512 w520 w530 w540] -> w454
          tunnel: [w493 w498 w508 w518 w528 w538] -> w453
          frame "False", Default {
            w493 = FALSE  # Visible
            w496 = FALSE  # Menu?
            n231 = local read "UI Output"() -> (w494:string)
          }
          frame "Main" {
            w498 = FALSE  # Visible
            w506 = TRUE  # Menu?
            n232 = Add(x=w501, y=5) -> (x+y=w503:i32)
            n233 = Bundle By Name(cluster=w500, "Left"=w502, "Top"=w503) -> (w499:T9)
          }
          frame "simulation" {
            w508 = TRUE  # Visible
            w516 = TRUE  # Menu?
            n234 = Add(x=w510, y=5) -> (x+y=w509:i32)
            n235 = Bundle By Name(cluster=w514, "Left"=w513, "Top"=w509) -> (w512:T9)
          }
          frame "ME" {
            w518 = TRUE  # Visible
            w526 = TRUE  # Menu?
            n236 = Add(x=w519, y=110) -> (x+y=w523:i32)
            n237 = Bundle By Name(cluster=w521, "Left"=w522, "Top"=w523) -> (w520:T9)
          }
          frame "User Utils" {
            w528 = TRUE  # Visible
            w536 = TRUE  # Menu?
            n238 = Add(x=w529, y=300) -> (x+y=w533:i32)
            n239 = Bundle By Name(cluster=w531, "Left"=w532, "Top"=w533) -> (w530:T9)
          }
          frame "Developer Tools" {
            w538 = TRUE  # Visible
            w546 = TRUE  # Menu?
            n240 = Add(x=w539, y=395) -> (x+y=w543:i32)
            n241 = Bundle By Name(cluster=w541, "Left"=w542, "Top"=w543) -> (w540:T9)
          }
        }
        n242 = case shown="False" w470 {
          tunnel: [w477 w484] -> w461
          tunnel: w468 -> [_ w486]
          tunnel: w467 -> [_ w490]
          tunnel: w471 -> [_ w487]
          tunnel: w469 -> [w478 _]
          tunnel: w458 -> [w475 w483]
          tunnel: w454 -> [_ w481]
          tunnel: w453 -> [_ w480]
          tunnel: w450 -> [_ w479]
          frame False {
            w476 = FALSE ("Visible")
            # "Not a menu Load a vi"
            n243 = One Button Dialog(message=w478) -> ()  [unwired: 1 in, 1 out]
            n244 = local write "SubmenuVisible"(w476) -> ()
            n245 = property on="ButtonsMenu" class="TabCtl (strict)"(error in=w475, "Visible"=w476) -> (error out=w477:errorcluster)  [unwired: 1 in, 1 out]
          }
          frame True {
            # "Menu"
            n246 = property on="Selector Panel" class="SubPnl"("Position"=w481, "Visible"=w480) -> ()  [unwired: 2 in, 2 out]
            n247 = call "GetVIPaths.vi"("MenuType"=w487, "error in (no error)"=w483) -> ("error out"=w492:errorcluster, "SubMenu VIs"=w489:path[], "Menu VIs"=w488:path[])  [unwired: 4 in]
            n248 = local read "SubmenuVisible"() -> (w482:bool)
            n249 = call "ButtonControl.vi"("SubPanel Command"=ButtonCommands."Load Buttons", "user event in"=w479, "MenuButtons"=w488, "error in (no error)"=w492, "SubMenuButtons"=w489, "SubMenuButtonPanels"=w490, "MenuButtonPanels"=w486) -> ("error out"=w485:errorcluster)  [unwired: 2 in, 1 out]
            n250 = property on="ButtonsMenu" class="TabCtl (strict)"(error in=w485, "Visible"=w482) -> (error out=w484:errorcluster)  [unwired: 1 in, 1 out]
          }
        }
        n251 = call "DeferPanelUpdates.vi"("error in (no error)"=w461, "Defer Panel Updates"=FALSE, "VI in"=w459) -> ("error out"=w460:errorcluster)  [unwired: 8 in]
      }
      frame "Sorting Submenu" {
        n252 = call "Set State Display.vi"("State"=w555, "error in (no error)"=w554) -> ("error out"=w551:errorcluster)  [unwired: 6 in]
        n253 = local read "UI Output"() -> (w549:string)
        n254 = case shown="\"False\", Default" w549 {
          tunnel: w551 -> [w557 w560]
          tunnel: [w557 w559] -> w550
          tunnel: [w556 SetupModeState."Exiting" ("State")] -> w548
          frame "False", Default {
            w556 = SetupModeState."Idling"  # State
          }
          frame "Close Screen" {
            n255 = property on="exit" class="Bool (strict)"(error in=w560, "Val(Sgnl)"=TRUE ("Value (Signaling)")) -> (error out=w559:errorcluster)  [unwired: 1 in, 1 out]
          }
        }
        n256 = local read "SubmenuVisible"() -> (w552:bool)
        n257 = property on="ButtonsMenu" class="TabCtl (strict)"(error in=w550, "Visible"=w552) -> (error out=w553:errorcluster)  [unwired: 1 in, 1 out]
      }
      frame "Resetting Menu" {
        w571 = SetupModeState."Sorting Menu"  # State
        n258 = call "DeferPanelUpdates.vi"("error in (no error)"=w566, "Defer Panel Updates"=TRUE, "VI in"=w564) -> ("error out"=w562:errorcluster)  [unwired: 8 in]
        n259 = call "ButtonControl.vi"("SubPanel Command"=ButtonCommands."Remove Buttons", "error in (no error)"=w562) -> ("error out"=w567:errorcluster)  [unwired: 7 in, 1 out]
        n260 = call <vilib>:"Clear Errors.vi"("error in (no error)"=w567) -> ("error out"=w563:errorcluster)  [unwired: 5 in, 1 out]
        n261 = call "DeferPanelUpdates.vi"("error in (no error)"=w563, "Defer Panel Updates"=FALSE, "VI in"=w564) -> ("error out"=w565:errorcluster)  [unwired: 8 in]
      }
      frame "Idling" {
        # "Transition"
        # "State"
        n262 = call "Set State Display.vi"("State"=w582, "error in (no error)"=w583) -> ("error out"=w577:errorcluster)  [unwired: 6 in]
        n263 = call "StateQ.vi"("QueueCommand"=QueueCommand."Get Ref", "error in (no error)"=w577) -> ("error out"=w579:errorcluster, "queue out"=w578:refnum<queue>)  [unwired: 5 in]
        n264 = Dequeue Element(queue=w578, error in (no error)=w579) -> (element=w581:T10, error out=w576:errorcluster)  [unwired: 1 in, 2 out]
        n265 = Unbundle By Name(w581) -> ("Transition"=w575:T11, "variant"=w572:variant)
        n266 = case shown="\"UI Button Pressed\"" w575 {
          tunnel: [SetupModeState."Idling" ("State 2") SetupModeState."Running" ("State 2") SetupModeState."Sorting Submenu" ("State 2") SetupModeState."Resetting Menu" ("State 2") SetupModeState."Erroring" ("State 2") SetupModeState."Exiting" ("State 2")] -> w573
          tunnel: w576 -> [w584 w586 w588 w590 _ w594]
          tunnel: [w584 w586 w588 w590 errorcluster {"status"=TRUE, "code"=99998, "source"="State Error"} ("error out") w594] -> w574
          tunnel: w572 -> [_ _ _ _ _ _]
          frame "No Transition - Error", Default {
            # "Can Trap This"
          }
          frame "Start" {
          }
          frame "UI Button Pressed" {
          }
          frame "Menu Button Pressed" {
          }
          frame "Generate Error" {
          }
          frame "Exit" {
          }
        }
      }
      frame "Running" {
        # "Transition"
        # "State"
        n267 = call "Set State Display.vi"("State"=w606, "error in (no error)"=w607) -> ("error out"=w601:errorcluster)  [unwired: 6 in]
        n268 = call "StateQ.vi"("QueueCommand"=QueueCommand."Get Ref", "error in (no error)"=w601) -> ("error out"=w603:errorcluster, "queue out"=w602:refnum<queue>)  [unwired: 5 in]
        n269 = Dequeue Element(queue=w602, error in (no error)=w603) -> (element=w605:T10, error out=w600:errorcluster)  [unwired: 1 in, 2 out]
        n270 = Unbundle By Name(w605) -> ("Transition"=w599:T11, "variant"=w596:variant)
        n271 = case shown="\"Stop\"" w599 {
          tunnel: [SetupModeState."Idling" ("State 2") SetupModeState."Idling" ("State 2") SetupModeState."Erroring" ("State 2") SetupModeState."Exiting" ("State 2")] -> w597
          tunnel: w600 -> [w608 w610 _ w614]
          tunnel: [w608 w610 errorcluster {"status"=TRUE, "code"=99998, "source"="State Error"} ("error out") w614] -> w598
          tunnel: w596 -> [_ _ _ _]
          frame "No Transition - Error", Default {
            # "Can Trap This"
          }
          frame "Stop" {
          }
          frame "Generate Error" {
          }
          frame "Exit" {
          }
        }
      }
      frame "Erroring" {
        # "Transition"
        # "State"
        n272 = call "Set State Display.vi"("State"=w616, "error in (no error)"=w620) -> ("error out"=w617:errorcluster)  [unwired: 6 in]
        n273 = call "WaitForTransition.vi"("error in (no error)"=w617, "State"=w616) -> ("error out"=w618:errorcluster, "StateOut"=w619:T1)  [unwired: 4 in]
      }
      frame "Exiting" {
        n274 = call "DeferPanelUpdates.vi"("error in (no error)"=w638, "Defer Panel Updates"=TRUE, "VI in"=w639) -> ("error out"=w642:errorcluster)  [unwired: 8 in]
        n275 = call "Set State Display.vi"("State"=w640, "error in (no error)"=w642) -> ("error out"=w635:errorcluster)  [unwired: 6 in]
        n276 = property on="ButtonsMenu" class="TabCtl (strict)"(error in=w635, "Visible"=FALSE) -> (error out=w634:errorcluster)  [unwired: 1 in, 1 out]
        n277 = call "ButtonControl.vi"("SubPanel Command"=ButtonCommands."Remove Buttons", "error in (no error)"=w634) -> ("error out"=w630:errorcluster)  [unwired: 7 in, 1 out]
        n278 = local read "BGND ref out"() -> (w628:refnum<vi>)
        n279 = invoke class="VI" method="Abort VI"(reference=w628, error in=w630) -> (error out=w633:errorcluster)  [unwired: 1 in, 2 out]
        n280 = control-ref of="Background"() -> (w629:refnum<vi>)
        n281 = call <vilib>:"Clear Errors.vi"("error in (no error)"=w633) -> ("error out"=w631:errorcluster)  [unwired: 5 in, 1 out]
        n282 = invoke on="Invoke Node" class="SubPnl" method="Remove VI"(reference=w629, error in=w631) -> (error out=w632:errorcluster)  [unwired: 1 in, 2 out]
        n283 = call <vilib>:"Clear Errors.vi"("error in (no error)"=w632) -> ("error out"=w624:errorcluster)  [unwired: 5 in, 1 out]
        n284 = local read "Selector ref out"() -> (w621:refnum<vi>)
        n285 = invoke class="VI" method="Abort VI"(reference=w621, error in=w624) -> (error out=w625:errorcluster)  [unwired: 1 in, 2 out]
        n286 = control-ref of="Selector Panel"() -> (w622:refnum<vi>)
        n287 = call <vilib>:"Clear Errors.vi"("error in (no error)"=w625) -> ("error out"=w627:errorcluster)  [unwired: 5 in, 1 out]
        n288 = invoke on="Invoke Node" class="SubPnl" method="Remove VI"(reference=w622, error in=w627) -> (error out=w626:errorcluster)  [unwired: 1 in, 2 out]
        n289 = call <vilib>:"Clear Errors.vi"("error in (no error)"=w626) -> ("error out"=w623:errorcluster)  [unwired: 5 in, 1 out]
        n290 = call "DeferPanelUpdates.vi"("error in (no error)"=w623, "Defer Panel Updates"=FALSE, "VI in"=w639) -> ("error out"=w637:errorcluster)  [unwired: 8 in]
      }
    }
    n291 = Format Into String(format string="%s", initial string="4.State Machine\n", w403) -> (resulting string=w402:string)  [unwired: 1 in, 1 out]
    n292 = call "Error Control.vi"("Command"=ErrorCommand."Set Error", "error in (no error)"=w404, "Source"=w402) -> ()  [unwired: 5 in, 1 out]
    "StateMachineLoop" <- w406
    "State" <- w403
  }
  n293 = while {
    tunnel: w21 -> [w657]
    tunnel: w22 -> [w656]
    tunnel: [w648] -> w9
    tunnel: [-1 ("ErrorHandlingLoop")] -> w28
    i -> [w650]
    stop <- w651 stop-if-true
    (unwired) DisplayMessage."No Message - Ignore" ("DisplayMessage")
    # "5. Error Handling"
    n294 = Dequeue Element(queue=w656, error in (no error)=w657) -> (element=w655:cluster{"ErrorMessage":T13, "DataIn":variant}, error out=w652:errorcluster)  [unwired: 1 in, 2 out]
    n295 = Unbundle By Name(w655) -> ("ErrorMessage"=w653:T13, "DataIn"=w654:variant)
    n296 = case shown="\"Display Message\"" w653 {
      tunnel: w654 -> [_ w674 _]
      tunnel: w652 -> [w658 w673 w677]
      tunnel: [w658 w664 w677] -> w648
      tunnel: [_ FALSE ("STOP?") TRUE ("STOP?")] -> w651
      tunnel: string[] [] -> [_ w672 _]
      frame "No Message - Ignore", Default {
        n297 = Wait (ms)(milliseconds to wait=u32 1) -> ()  [unwired: 1 out]
      }
      frame "Display Message" {
        n298 = Variant To Data(error in=w673, type=w672, Variant=w674) -> (data=w666:string[], error out=w665:errorcluster)
        n299 = Get Date/Time String(date format (0)=enum16{"short", "long", "abbreviated"}."short", want seconds? (F)=TRUE) -> (date string=w669:string, time string=w668:string)  [unwired: 1 in]
        n300 = Concatenate Strings(w669, " " ("string"), w668) -> (w660:string)
        "Error" <- w660
        n301 = Build Array (concatenate)(w660, w666) -> (w661:string[])
        n302 = call "DisplayQ.vi"("command"=DisplayQCommand."Add Item to Bottom", "error in (no error)"=w665, "DataIn"=w661, "DisplayMessage"=DisplayMessage."Add Error Message") -> ("error out"=w664:errorcluster)  [unwired: 1 in, 3 out]
      }
      frame "Stop" {
      }
    }
    "ErrorHandlingLoop" <- w650
  }
  n303 = local write "ErrorHandlingLoop"(w28) -> ()
  n304 = call "DisplayQ.vi"("command"=DisplayQCommand."Close", "error in (no error)"=w9) -> ("error out"=w11:errorcluster)  [unwired: 3 in, 3 out]
  n305 = call "StateQ.vi"("QueueCommand"=QueueCommand."Close", "error in (no error)"=w11) -> ("error out"=w13:errorcluster)  [unwired: 5 in, 1 out]
  n306 = call "ErrorQ.vi"("command"=DisplayQCommand."Close", "error in (no error)"=w13) -> ("error out"=w14:errorcluster)  [unwired: 3 in, 3 out]
  n307 = call "SSDCExit.vi"("error in (no error)"=w14) -> ()  [unwired: 6 in, 1 out]
  n308 = local write "UILoop"(w26) -> ()
  n309 = local write "EventLoop"(w25) -> ()
  n310 = local write "StateMachineLoop"(w27) -> ()
